vi "Check-Batch-selector.vi"(8 "error in":errorcluster, 10 "Acquis. params. ref.":refnum<data-value>, 11 "Batch browser":refnum<vi>) -> (0 "error IO":errorcluster, 1 "Time selector value":i32, 2 "Batch size":i32, 3 "Time selector minimum":dbl)   [LabVIEW 2013, in "CameraVision.lvlib" / "CV-UI.lvclass"]
doc: "This function adapts the limits and value of the 'Batch browser' front panel control according to the acquisition parameters."
uses:
  CV-UI.lvclass
  Main/Acquisition/CV-Acquisition.lvclass
  Main/Acquisition/CV-Acquisition.lvclass/CV-Acquisition.ctl
  Main/Acquisition/Read Acquisition mode.vi
  Main/Acquisition/Read Batch size.vi
  Main/Acquisition/Write Batch size var.vi
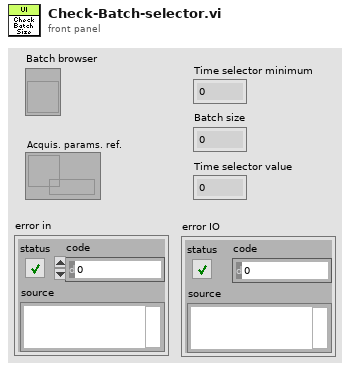
[diagram p1: front panel]
types:
  T1 = enum8{"Enabled", "Disabled", "Disabled and Grayed Out"}
  T2 = enum16{"Continuous", "Continuous batch", "Single batch", "Single batch -delayed"}
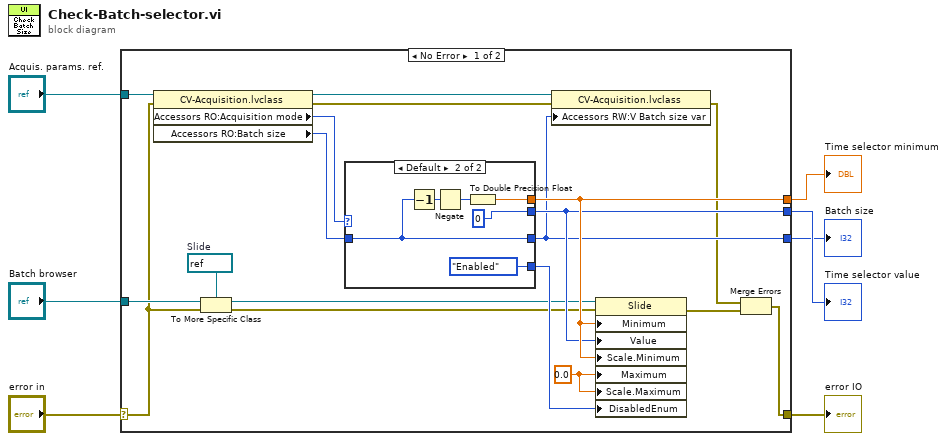
[diagram p0: block diagram]
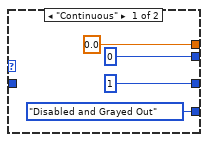
[diagram p2: hidden frame]
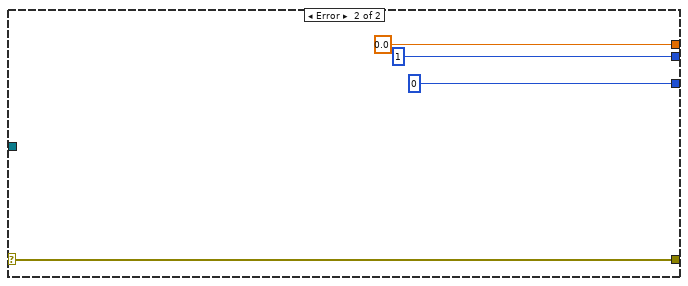
[diagram p3: hidden frame]
diagram:
  n1 = case shown="No Error" "error in" {
    selector: "error in" -> [w10 w38]
    tunnel: [w24 0.0 ("Batch size")] -> w7
    tunnel: [w23 1] -> w6
    tunnel: [w16 w38] -> w4
    tunnel: [w14 0 ("Batch size")] -> w3
    tunnel: "Batch browser" -> [w20 _]
    tunnel: "Acquis. params. ref." -> [w19 _]
    frame No Error {
      w8 = refnum<vi> refnum  # Slide
      w25 = 0.0 ("Data Entry Limits:Maximum")
      n2 = property class="CV-Acquisition.lvclass"(reference=w19, error in=w10) -> (reference out=w15:refnum<data-value>, error out=w12:errorcluster, "Accessors RO:Acquisition mode"=w18:T2, "Accessors RO:Batch size"=w17:i32)
      n3 = To More Specific Class(target class=w8, reference=w20, error in=w10) -> (specific class reference=w11:refnum<vi>, error out=w9:errorcluster)
      n4 = case shown="Default" w18 {
        tunnel: w17 -> [_ w33]
        tunnel: [0.0 ("Batch size") w31] -> w24
        tunnel: [0 0] -> w23
        tunnel: [1 ("Batch size") w33] -> w14
        tunnel: [T1."Disabled and Grayed Out" ("Disabled") T1."Enabled" ("Disabled")] -> w21
        frame "Continuous" {
        }
        frame Default {
          n5 = Decrement(x=w33) -> (x-1=w32:i32)
          n6 = Negate(x=w32) -> (-x=w34:i32)
          n7 = To Double Precision Float(number=w34) -> (double precision float=w31:dbl)
        }
      }
      n8 = property class="CV-Acquisition.lvclass"(reference=w15, error in=w12, "Accessors RW:V Batch size var"=w14) -> (error out=w13:errorcluster)  [unwired: 1 out]
      n9 = property on="Property Node" class="Slide"(reference=w11, error in=w9, "Minimum"=w24, "Value"=w23, "Scale.Minimum"=w24, "Maximum"=w25, "Scale.Maximum"=w25, "DisabledEnum"=w21) -> (error out=w22:errorcluster)  [unwired: 1 out]
      n10 = Merge Errors(w13, w22) -> (w16:errorcluster)
    }
    frame Error {
    }
  }
  "Time selector minimum" <- w7
  "Time selector value" <- w6
  "error IO" <- w4
  "Batch size" <- w3
